vi "Lvdt data.vi"(11 "Lvdt":refnum<vi>) -> (0 "LVDT":bool, 1 "lvdt":dbl, 2 "lvdt":dbl format="%0.03f")   [LabVIEW 2015]
uses:
  Galobal variable_TI.vi
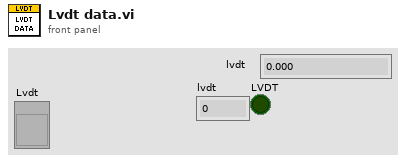
[diagram p1: front panel]
types:
  T1 = cluster{"MaxLoad(N) ":dbl, "Min Load(N)":dbl, "Load Offset":dbl, "Model":string, "MIC Code":string, "Dial Speedo":string, "Dial RMP":string, "Blinker":string, "Telltale":string}
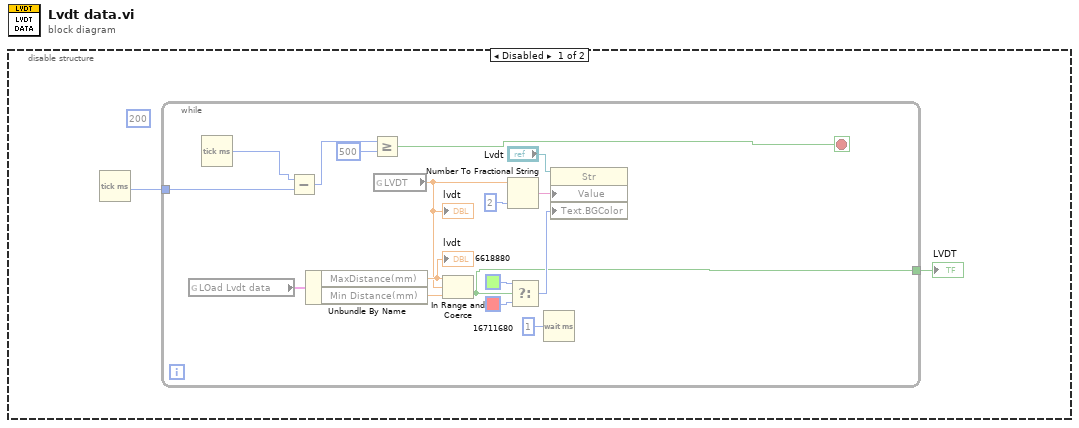
[diagram p0: block diagram]
diagram:
  n1 = disable-structure shown="Disabled" {
    frame Disabled {
      (unwired) 200
      n2 = Tick Count (ms)() -> (millisecond timer value=w2:u32)
      n3 = while {
        tunnel: w2 -> [w8]
        tunnel: [w3] -> w1
        stop <- w5 stop-if-true
        n4 = global read "Galobal variable_TI.vi" "LOad Lvdt data"() -> (w13:T1)
        n5 = Tick Count (ms)() -> (millisecond timer value=w9:u32)
        n6 = Subtract(x=w9, y=w8) -> (x-y=w7:u32)
        n7 = Unbundle By Name(w13) -> ("MaxDistance(mm)"=w12:dbl, "Min Distance(mm)"=w11:dbl)
        "lvdt" <- w12
        n8 = Greater Or Equal?(x=w7, y=u32 500) -> (x >= y?=w5:bool)
        n9 = global read "Galobal variable_TI.vi" "LVDT"() -> (w10:dbl)
        "lvdt" <- w10
        n10 = In Range and Coerce(upper limit=w12, x=w10, lower limit=w11) -> (In Range?=w3:bool)  [unwired: 1 out]
        n11 = Number To Fractional String(number=w10, precision (6)=i16 2) -> (F-format string=w16:string)  [unwired: 2 in]
        n12 = Select(t=u32 6618880, s=w3, f=u32 16711680) -> (s? t:f=w19:u32)
        n13 = Wait (ms)(milliseconds to wait=u32 1) -> ()  [unwired: 1 out]
        n14 = property class="Str"(reference="Lvdt", "Value"=w16, "Text.BGColor"=w19) -> ()  [unwired: 1 in, 2 out]
      }
      "LVDT" <- w1
    }
    frame Enabled {
    }
  }
